vi "WriteReadN-ver4.vi"() -> ()   [LabVIEW 2014]
uses:
  (Global) Current handle and LaserPower_YCC.vi
panel:
  in  "milliseconds to wait":u32=500
  out "Current Position Z (um)":dbl format="%.4f"
  out "Current Position Y (um)":dbl format="%.4f"
  out "Current Position X (um)":dbl format="%.4f"
  in  "read #":i32=1
  in  "Z Move to (um)":dbl=50.0 format="%_6g"
  in  "Y Move to (um)":dbl=50.0 format="%_6g"
  in  "X Move to (um)":dbl=50.0 format="%_6g"
  in  "Chang Z?":bool
  in  "Chang Y?":bool
  in  "Chang X?":bool
  in  "Reset ? (move to (50,50,50))":bool=TRUE
  in  "turn off stage":bool
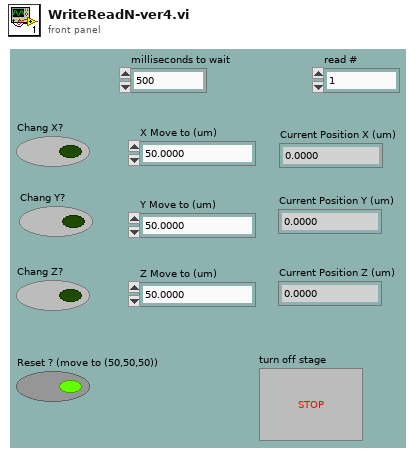
[diagram p1: front panel]
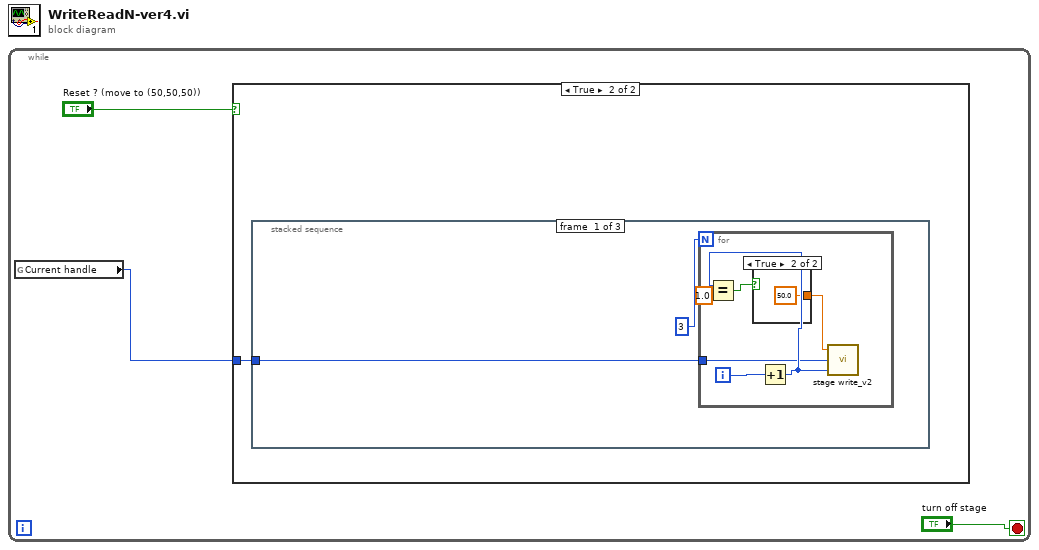
[diagram p0: block diagram]
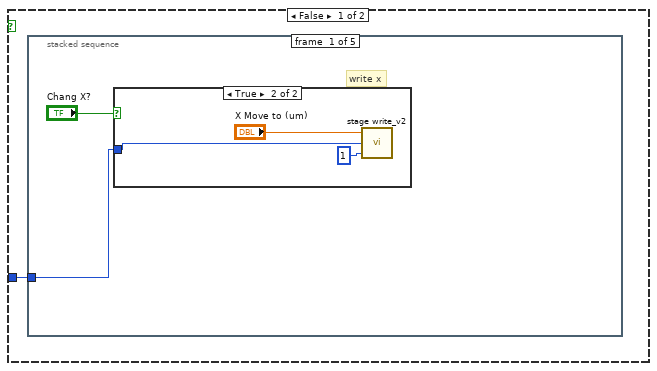
[diagram p2: hidden frame]
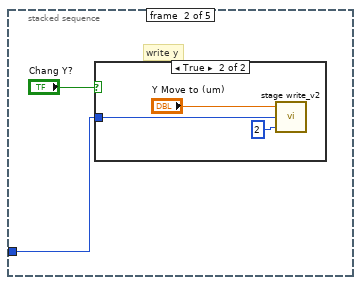
[diagram p4: hidden frame]
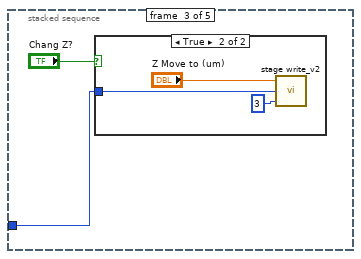
[diagram p6: hidden frame]
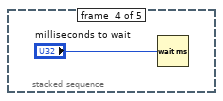
[diagram p8: hidden frame]
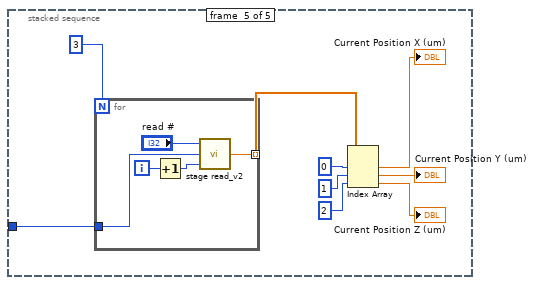
[diagram p9: hidden frame]
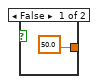
[diagram p10: hidden frame]
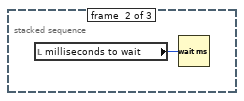
[diagram p11: hidden frame]
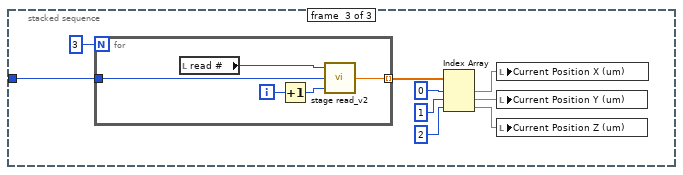
[diagram p12: hidden frame]
diagram:
  n1 = while {
    stop <- "turn off stage" stop-if-true
    n2 = global read "(Global) Current handle and LaserPower_YCC.vi" "Current handle"() -> (w1:i32)
    n3 = case shown="True" "Reset ? (move to (50,50,50))" {
      tunnel: w1 -> [w4 w35]
      frame False {
        n4 = stacked-sequence {
          tunnel: w4 -> [w5 w10 w15 _ w21]
          frame #0 {
            # "write x"
            n5 = case shown="True" "Chang X?" {
              tunnel: w5 -> [_ w7]
              frame False {
              }
              frame True {
                n6 = call "stage write_v2.vi"("axis"=u32 1, "Incoming Handle"=w7, "position"="X Move to (um)") -> ()  [unwired: 2 in, 1 out]
              }
            }
          }
          frame #1 {
            # "write y"
            n7 = case shown="True" "Chang Y?" {
              tunnel: w10 -> [_ w12]
              frame False {
              }
              frame True {
                n8 = call "stage write_v2.vi"("axis"=u32 2, "Incoming Handle"=w12, "position"="Y Move to (um)") -> ()  [unwired: 2 in, 1 out]
              }
            }
          }
          frame #2 {
            n9 = case shown="True" "Chang Z?" {
              tunnel: w15 -> [_ w17]
              frame False {
              }
              frame True {
                n10 = call "stage write_v2.vi"("axis"=u32 3, "Incoming Handle"=w17, "position"="Z Move to (um)") -> ()  [unwired: 2 in, 1 out]
              }
            }
          }
          frame #3 {
            n11 = Wait (ms)(milliseconds to wait="milliseconds to wait") -> ()  [unwired: 1 out]
          }
          frame #4 {
            n12 = for {
              N: 3 -> [_]
              tunnel: [w31] -> w28 mode=indexing
              tunnel: w21 -> [w30]
              i -> [w34]
              n13 = Increment(x=w34) -> (x+1=w33:i32)
              n14 = call "stage read_v2.vi"("Axis"=w33, "Incoming Handle"=w30, "read #"="read #") -> ("position (um)"=w31:dbl)  [unwired: 1 in, 1 out]
            }
            n15 = Index Array(array=w28, index #1=0 ("index"), index #2=1 ("index"), index #3=2 ("index")) -> (element #1=→"Current Position X (um)":dbl, element #2=→"Current Position Y (um)":dbl, element #3=→"Current Position Z (um)":dbl)
          }
        }
      }
      frame True {
        n16 = stacked-sequence {
          tunnel: w35 -> [w36 _ w47]
          frame #0 {
            n17 = for {
              N: 3 -> [_]
              tunnel: w36 -> [w38]
              i -> [w43]
              n18 = Increment(x=w43) -> (x+1=w40:i32)
              n19 = Equal?(x=w40, y=1.0) -> (x = y?=w39:bool)
              n20 = case shown="True" w39 {
                tunnel: [50.0 ("position") 50.0 ("position")] -> w42
                frame False {
                }
                frame True {
                }
              }
              n21 = call "stage write_v2.vi"("axis"=w40, "Incoming Handle"=w38, "position"=w42) -> ()  [unwired: 2 in, 1 out]
            }
          }
          frame #1 {
            n22 = local read "milliseconds to wait"() -> (w46:u32)
            n23 = Wait (ms)(milliseconds to wait=w46) -> ()  [unwired: 1 out]
          }
          frame #2 {
            n24 = for {
              N: 3 -> [_]
              tunnel: [w58] -> w54 mode=indexing
              tunnel: w47 -> [w56]
              i -> [w60]
              n25 = local read "read #"() -> (w57:i32)
              n26 = Increment(x=w60) -> (x+1=w59:i32)
              n27 = call "stage read_v2.vi"("Axis"=w59, "Incoming Handle"=w56, "read #"=w57) -> ("position (um)"=w58:dbl)  [unwired: 1 in, 1 out]
            }
            n28 = Index Array(array=w54, index #1=0 ("index"), index #2=1 ("index"), index #3=2 ("index")) -> (element #1=w50:dbl, element #2=w49:dbl, element #3=w48:dbl)
            n29 = local write "Current Position X (um)"(w50) -> ()
            n30 = local write "Current Position Y (um)"(w49) -> ()
            n31 = local write "Current Position Z (um)"(w48) -> ()
          }
        }
      }
    }
  }
